vi "Get Temp Setpoint--Method.vi"(8 "error in (no error)":errorcluster, 10 "Temp Setpoint Data":T1, 11 "Watlow F4T in":refnum<class "Watlow F4T.lvclass">) -> (0 "error out":errorcluster, 1 "Actual Temp Setpoint":dbl, 2 "Target Temp Setpoint":dbl, 3 "Watlow F4T out":refnum<class "Watlow F4T.lvclass">)   [LabVIEW 2024, in "Watlow F4T.lvclass"]
uses:
  Watlow F4T.lvclass
  Process Controller/Controls/Temp Data--Cluster.ctl
  Process Controller/Controls/Temperature Units--Enum.ctl
  Process Controller/_Thermal Process Controller.lvclass
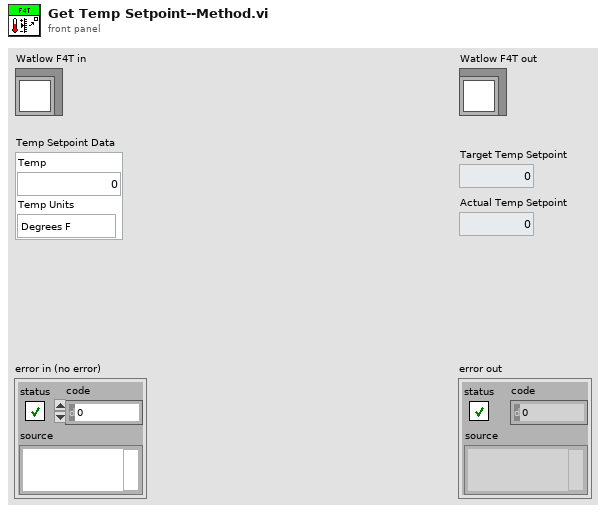
[diagram p1: front panel]
types:
  T1 = typedef "_Thermal Process Controller.lvclass/Temp Data--Cluster.ctl" = cluster{"Temp":dbl, "Temp Units":T2}
  T2 = typedef "_Thermal Process Controller.lvclass/Temperature Units--Enum.ctl" = enum16{"Degrees F", "Degrees C", "Degrees K"}
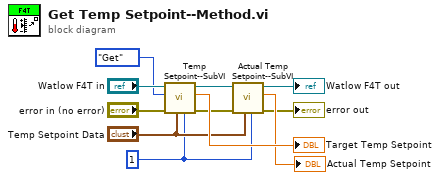
[diagram p0: block diagram]
diagram:
  w3 = 1 ("Instance(1)")
  n1 = call "Temp Setpoint--SubVI.vi"("Instance(1)"=w3, "Temp Setpoint Data"="Temp Setpoint Data", "error in (no error)"="error in (no error)", "Get/Set"=enum16{"Get", "Set"}."Get", "Watlow F4T In"="Watlow F4T in") -> ("error out"=w7:errorcluster, "Target Temp Setpoint"=→"Target Temp Setpoint":dbl, "Watlow F4T out"=w6:refnum<class "Watlow F4T.lvclass">)  [unwired: 4 in]
  n2 = call "Actual Temp Setpoint--SubVI.vi"("Instance(1)"=w3, "Temp Setpoint Data"="Temp Setpoint Data", "error in (no error)"=w7, "Watlow F4T In"=w6) -> ("error out"=→"error out":errorcluster, "Actual Temp Setpoint"=→"Actual Temp Setpoint":dbl, "Watlow F4T out"=→"Watlow F4T out":refnum<class "Watlow F4T.lvclass">)  [unwired: 5 in]
